vi "SPI Write Read.vi"(4 "CS Logic Level":T1, 6 "CS Pin (10)":u8=10, 7 "SPI Frame Size (1)":u8=1, 8 "Error In":errorcluster, 9 "Data":u8[](array[numeric]), 10 "SPI Channel":u8, 11 "LINX Device Config":T2) -> (0 "Error Out":errorcluster, 1 "Read Data":u8[](array[numeric]), 3 "LINX Device Config":T2)   [LabVIEW 2014, in "LMH-LINX.lvlib" / "Device.lvlib"]
doc: "Write/Read the specified SPI channel."
uses:
  <vilib>/MakerHub/LINX/Private/Device/Device.lvlib
  <vilib>/MakerHub/LINX/Private/Device/Type Defs/LINX Device Config.ctl
  <vilib>/MakerHub/LINX/Private/Type Defs/Interface.ctl
  <vilib>/MakerHub/LINX/Private/Device/Type Defs/TCP Config.ctl
  <vilib>/MakerHub/LINX/Private/Device/Type Defs/Channels.ctl
  <vilib>/MakerHub/LINX/Private/Type Defs/Peripherals/SPI/SPI CS Logic Level.ctl
  <vilib>/MakerHub/LINX/Private/Type Defs/Error Type.ctl
  <vilib>/MakerHub/LINX/LMH-LINX.lvlib
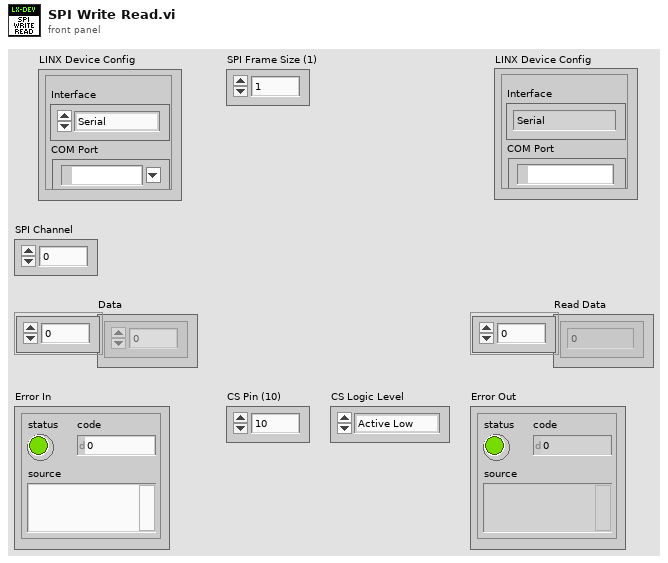
[diagram p1: front panel]
types:
  T1 = typedef "LMH-LINX.lvlib/SPI CS Logic Level.ctl" = enum8{"Active Low", "Active High"}
  T2 = typedef "LMH-LINX.lvlib/Device.lvlib/LINX Device Config.ctl" = cluster{"Interface":T3, "COM Port":refnum<visa-resource-name>, "TCP Configuration":T4, "Device Family":u8, "Device ID":u8, "Device Name":string, "TCP Ref":refnum<k5>, "Channels":T5}
  T3 = typedef "LMH-LINX.lvlib/Interface.ctl" = enum16{"Serial", "TCP"}
  T4 = typedef "LMH-LINX.lvlib/Device.lvlib/TCP Config.ctl" = cluster{"IP Address":string, "Port":u16}
  T5 = typedef "LMH-LINX.lvlib/Channels.ctl" = cluster{"DI":u8[], "DO":u8[], "AI":u8[], "AO":u8[], "PWM":u8[], "QE":u8[], "UART":u8[], "I2C 2":u8[], "SPI":u8[], "CAN":u8[], "Servo":u8[], "AI Ref (V)":dbl, "AI Resolution (Bits)":u8, "AO Ref (V)":dbl, "AO Resolution (Bits)":u8}
  T6 = typedef "LMH-LINX.lvlib/Error Type.ctl" = enum16{"Unknown", "Timeout", "Corrupt Return Packet", "Unable To Connect", "Command Not Supported", "Channel DNE", "Invalid COM Config", "Firmware Version Mismatch", "myRIO Support", "CMD Specific Error", "Local IO Not Supported"}
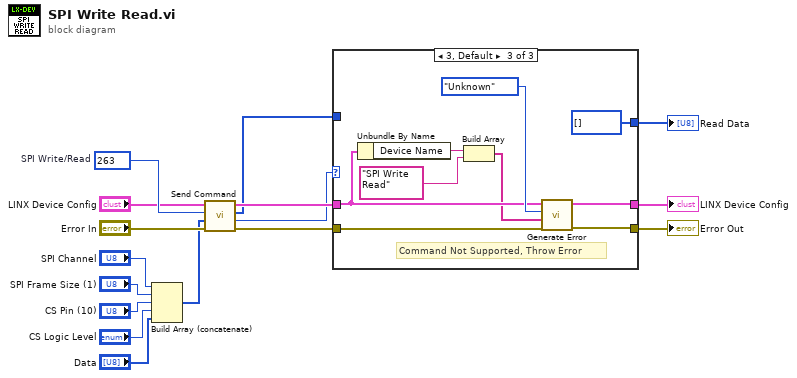
[diagram p0: block diagram]
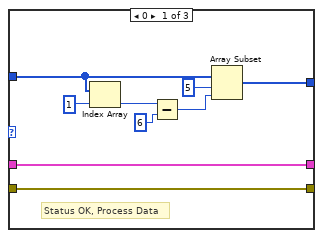
[diagram p2: hidden frame]
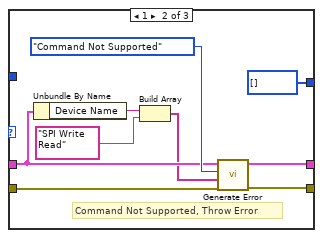
[diagram p3: hidden frame]
diagram:
  w15 = u16 263  # SPI Write/Read
  n1 = Build Array (concatenate)("SPI Channel", "SPI Frame Size (1)", "CS Pin (10)", "CS Logic Level", "Data") -> (w8:u8[])
  n2 = call <vilib>:"Send Command.vi"("Error In"="Error In", "ARGS"=w8, "CMD"=w15, "LINX Device Config"="LINX Device Config") -> ("Error Out"=w10:errorcluster, "Status"=w1:u8, "Response"=w7:u8[], "LINX Device Config"=w12:T2)  [unwired: 4 in]
  n3 = case shown="3, Default" w1 {
    tunnel: [w25 w32 w41] -> w13
    tunnel: w12 -> [w25 w28 w37]
    tunnel: [w24 w33 w42] -> w11
    tunnel: w10 -> [w24 w34 w43]
    tunnel: w7 -> [w17 _ _]
    tunnel: [w20 u8[] [] u8[] []] -> w6
    frame 0 {
      # "Status OK, Process Data"
      n4 = Index Array(array=w17, index=1) -> (element=w18:u8)
      n5 = Subtract(x=w18, y=u8 6) -> (x-y=w22:u8)
      n6 = Array Subset(array=w17, index=5, length=w22) -> (w20:u8[])
    }
    frame 1 {
      # "Command Not Supported, Throw Error"
      n7 = Unbundle By Name(w28) -> ("Device Name"=w30:string)
      n8 = Build Array(w30, "SPI Write Read") -> (w27:string[])
      n9 = call <vilib>:"Generate Error.vi"("Error In"=w34, "Arguments"=w27, "Error Type"=Error_Type."Command Not Supported", "LINX Device Config"=w28) -> ("Error Out"=w33:errorcluster, "Dup LINX Device Config"=w32:T2)  [unwired: 6 in]
    }
    frame 3, Default {
      # "Command Not Supported, Throw Error"
      n10 = Unbundle By Name(w37) -> ("Device Name"=w39:string)
      n11 = Build Array(w39, "SPI Write Read") -> (w36:string[])
      n12 = call <vilib>:"Generate Error.vi"("Error In"=w43, "Arguments"=w36, "Error Type"=Error_Type."Unknown", "LINX Device Config"=w37) -> ("Error Out"=w42:errorcluster, "Dup LINX Device Config"=w41:T2)  [unwired: 6 in]
    }
  }
  "Error Out" <- w11
  "LINX Device Config" <- w13
  "Read Data" <- w6
